vi "Sequence Tester.vi"() -> ()   [LabVIEW 2014]
uses:
  DriverMasterSync/build/DriverMasterSync.lvlibp/Modules/HAL/DriverMasterSync/DriverMasterSyncClass/DriverMasterSync.lvclass
  <vilib>/Utility/LVLibp/NI_PackedLibraryUtility.lvlib
panel:
  out "TDX":sgl[][](array[numeric])
  in  "stop":bool
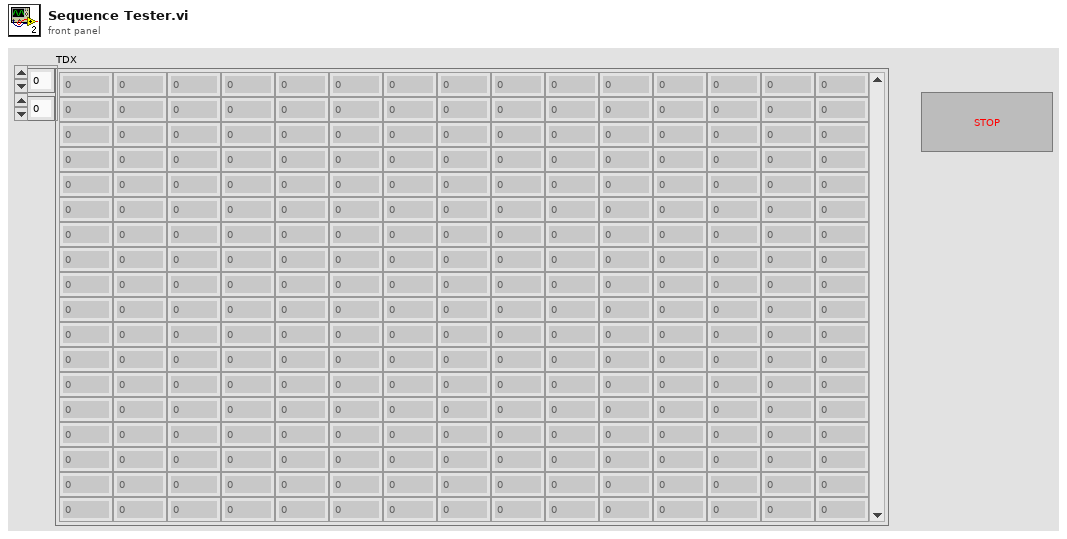
[diagram p1: front panel]
types:
  T1 = typedef "DriverMasterSync.lvlibp/WINFAS 2 Data Queue.lvlib/Control Data Cluster.ctl" = cluster{"Encoder":sgl, "DI":bool[], "DO":bool[]}
  T2 = typedef "DriverMasterSync.lvlibp/WINFAS 2 Data Queue.lvlib/Acquisition Data Cluster.ctl" = T3[]
  T3 = typedef "DriverMasterSync.lvlibp/WINFAS 2 Data Queue.lvlib/Acquisition Data 1 Sample Cluster.ctl" = cluster{"TDX":sgl[], "Encoder":sgl}
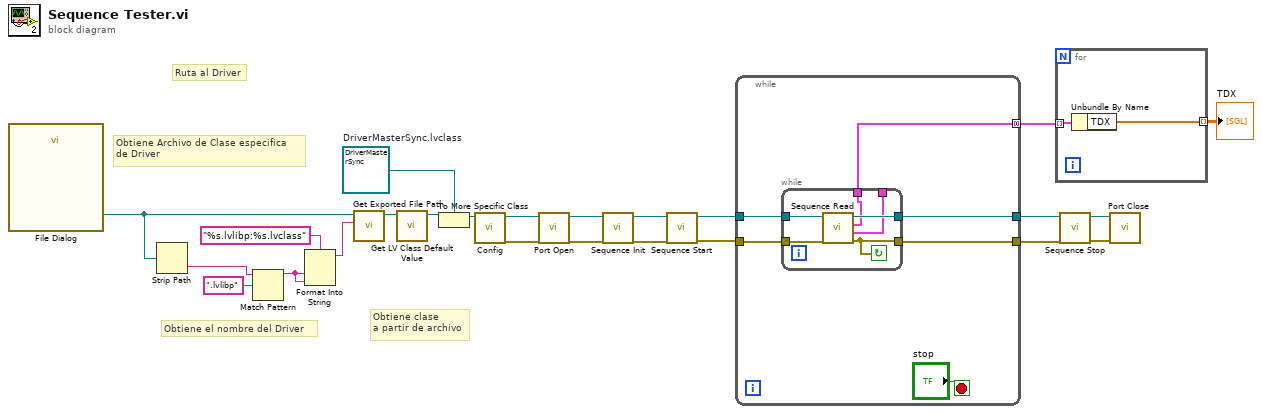
[diagram p0: block diagram]
diagram:
  w8 = refnum<class "DriverMasterSync.lvclass"> refnum  # DriverMasterSync.lvclass
  # "Ruta al Driver"
  # "Obtiene el nombre del Driver"
  # "Obtiene clase\na partir de archivo"
  # "Obtiene Archivo de Clase especifica\nde Driver"
  n1 = call "File Dialog"() -> ("selected path"=w4:path)  [unwired: 12 in, 3 out]
  n2 = Strip Path(path=w4) -> (name=w6:string)  [unwired: 1 out]
  n3 = Match Pattern(string=w6, regular expression=".lvlibp") -> (before substring=w5:string)  [unwired: 1 in, 3 out]
  n4 = Format Into String(format string="%s.lvlibp:%s.lvclass", w5, w5) -> (resulting string=w11:string)  [unwired: 2 in, 1 out]
  n5 = call <vilib>:"Get Exported File Path.vi"("qualified name"=w11, "packed library path"=w4) -> ("path"=w12:path)  [unwired: 8 in, 1 out]
  n6 = call <vilib>:"Get LV Class Default Value.vi"("class path"=w12) -> ("object"=w10:refnum<class>)  [unwired: 9 in, 1 out]
  n7 = To More Specific Class(target class=w8, reference=w10) -> (specific class reference=w3:refnum<class "DriverMasterSync.lvclass">)  [unwired: 1 in, 1 out]
  n8 = call-dynamic "Config.vi"("DriverMasterSync in"=w3) -> ("error out"=w18:errorcluster, "DriverMasterSync out"=w24:refnum<class "DriverMasterSync.lvclass">)  [unwired: 8 in, 1 out]
  n9 = call-dynamic "Port Open.vi"("error in (no error)"=w18, "DriverMasterSync in"=w24) -> ("error out"=w17:errorcluster, "DriverMasterSync out"=w23:refnum<class "DriverMasterSync.lvclass">)  [unwired: 8 in]
  n10 = call-dynamic "Sequence Init.vi"("error in (no error)"=w17, "DriverMasterSync in"=w23) -> ("error out"=w16:errorcluster, "DriverMasterSync out"=w22:refnum<class "DriverMasterSync.lvclass">)  [unwired: 8 in]
  n11 = call-dynamic "Sequence Start.vi"("error in (no error)"=w16, "DriverMasterSync in"=w22) -> ("error out"=w15:errorcluster, "DriverMasterSync out"=w21:refnum<class "DriverMasterSync.lvclass">)  [unwired: 8 in]
  n12 = while {
    tunnel: w15 -> [w28]
    tunnel: [w27] -> w14
    tunnel: w21 -> [w30]
    tunnel: [w29] -> w20
    tunnel: [w25] -> w2 mode=concatenating
    stop <- "stop" stop-if-true
    n13 = while {
      tunnel: [w32] -> _
      tunnel: w28 -> [w34]
      tunnel: [w33] -> w27
      tunnel: w30 -> [w36]
      tunnel: [w35] -> w29
      tunnel: [w31] -> w25
      stop <- w33 continue-if-true
      n14 = call-dynamic "Sequence Read.vi"("error in (no error)"=w34, "DriverMasterSync in"=w36) -> ("error out"=w33:errorcluster, "Control Data"=w32:T1, "Acquisition Data"=w31:T2, "DriverMasterSync out"=w35:refnum<class "DriverMasterSync.lvclass">)  [unwired: 6 in]
    }
  }
  n15 = for {
    tunnel: w2 -> [w38] mode=indexing
    tunnel: [w37] -> w1 mode=indexing
    n16 = Unbundle By Name(w38) -> ("TDX"=w37:sgl[])
  }
  "TDX" <- w1
  n17 = call-dynamic "Sequence Stop.vi"("error in (no error)"=w14, "DriverMasterSync in"=w20) -> ("error out"=w13:errorcluster, "DriverMasterSync out"=w19:refnum<class "DriverMasterSync.lvclass">)  [unwired: 8 in]
  n18 = call-dynamic "Port Close.vi"("error in (no error)"=w13, "DriverMasterSync in"=w19) -> ()  [unwired: 8 in, 2 out]
